vi "ScanMode_SLM.vi"() -> ()   [LabVIEW 2014]
uses:
  Controls/Scan_SLM.ctl
  Controls/MetricControl_SLM.ctl
  Controls/Scan Metric_SLM.ctl
  Controls/ScanEngineState_SLM.ctl
  <vilib>/Analysis/6fits.llb/Curve Fitting Criteria.ctl
  <vilib>/Utility/miscctls.llb/LVPointDoubleTypeDef.ctl
  <vilib>/Analysis/NI_AALPro.lvlib
  <vilib>/gmath/NI_Gmath.lvlib
panel:
  in  "Reset":bool
  out "Image":sgl[][](graph)
  in  "Apply":bool
  in  "Find peak":bool
  in  "Cancel":bool
  in  "Metric Control":T1
  in  "stop":bool
  out "Metric Display":cluster{"Amplititude":dbl[], "Metric":dbl[]}[](graph)
  in  "Scan Control":T3 {"Mode" items=["2", "3", "4", "5", "6", "7", "8", "9", "10", "11", "12", "13", "14", "15", "16", "17", "18", "19", "20", "21", "22", "23", "24", "25", "26", "27", "28", "29", "30", "31", "32", "33", "34", "35", "36", "37"]}
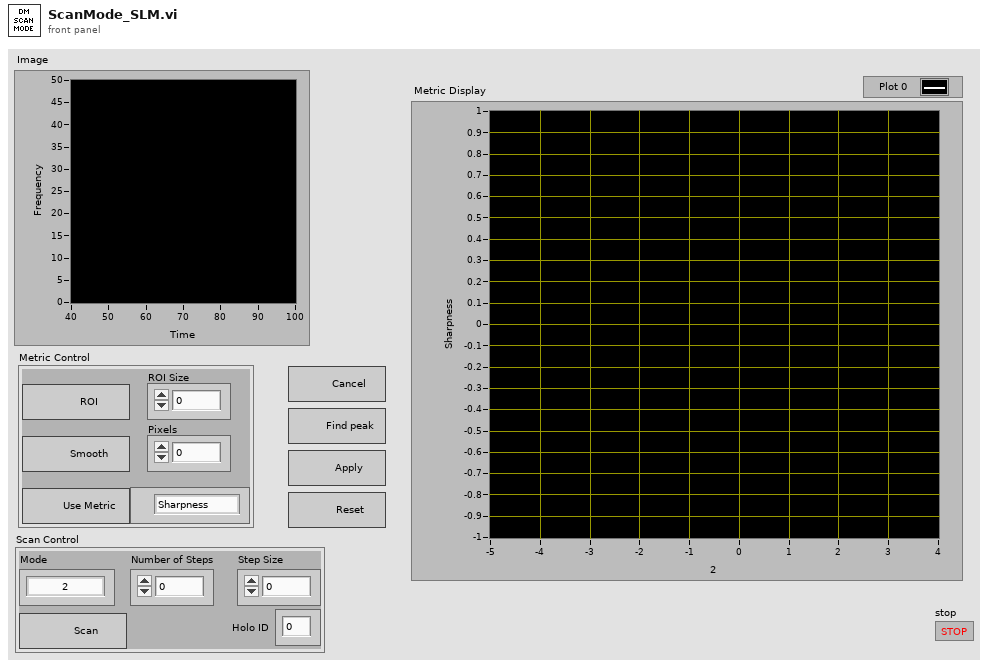
[diagram p1: front panel]
types:
  T1 = typedef "MetricControl_SLM.ctl" = cluster{"Use Metric":bool, "SLM Metric":T2, "Smooth":bool, "Pixels":dbl, "ROI":bool, "ROI Size":dbl}
  T2 = typedef "Scan Metric_SLM.ctl" = enum16{"Sharpness", "Brightness", "Combined"}
  T3 = typedef "Scan_SLM.ctl" = cluster{"Scan":bool, "Mode":u16, "Number of Steps":u8, "Step Size":dbl, "Holo ID":i32}
  T4 = typedef "ScanEngineState_SLM.ctl" = enum16{"SLM_WRITE", "IMAGE", ""}
  T5 = typedef "LVPointDoubleTypeDef.ctl" = cluster{"X":dbl, "Y":dbl}
  T6 = enum16{"Linear", "Polynomial", "Exponential", "Power"}
  T7 = typedef "Holo Settings.ctl" = cluster{"Top Hat":bool, "Modes":cluster{"Mode ID":string, "Amplititute":dbl}[], "Vortex":bool, "Clockwise":bool, "X":dbl, "Y":dbl, "Holo ON":bool, "Scan":bool}
  T8 = typedef "LVStringsAndValuesArrayTypeDef_U16.ctl" = cluster{"String":string, "Value":u16}[]
  T9 = typedef "NI_AALPro.lvlib/Curve Fitting Criteria.ctl" = u16
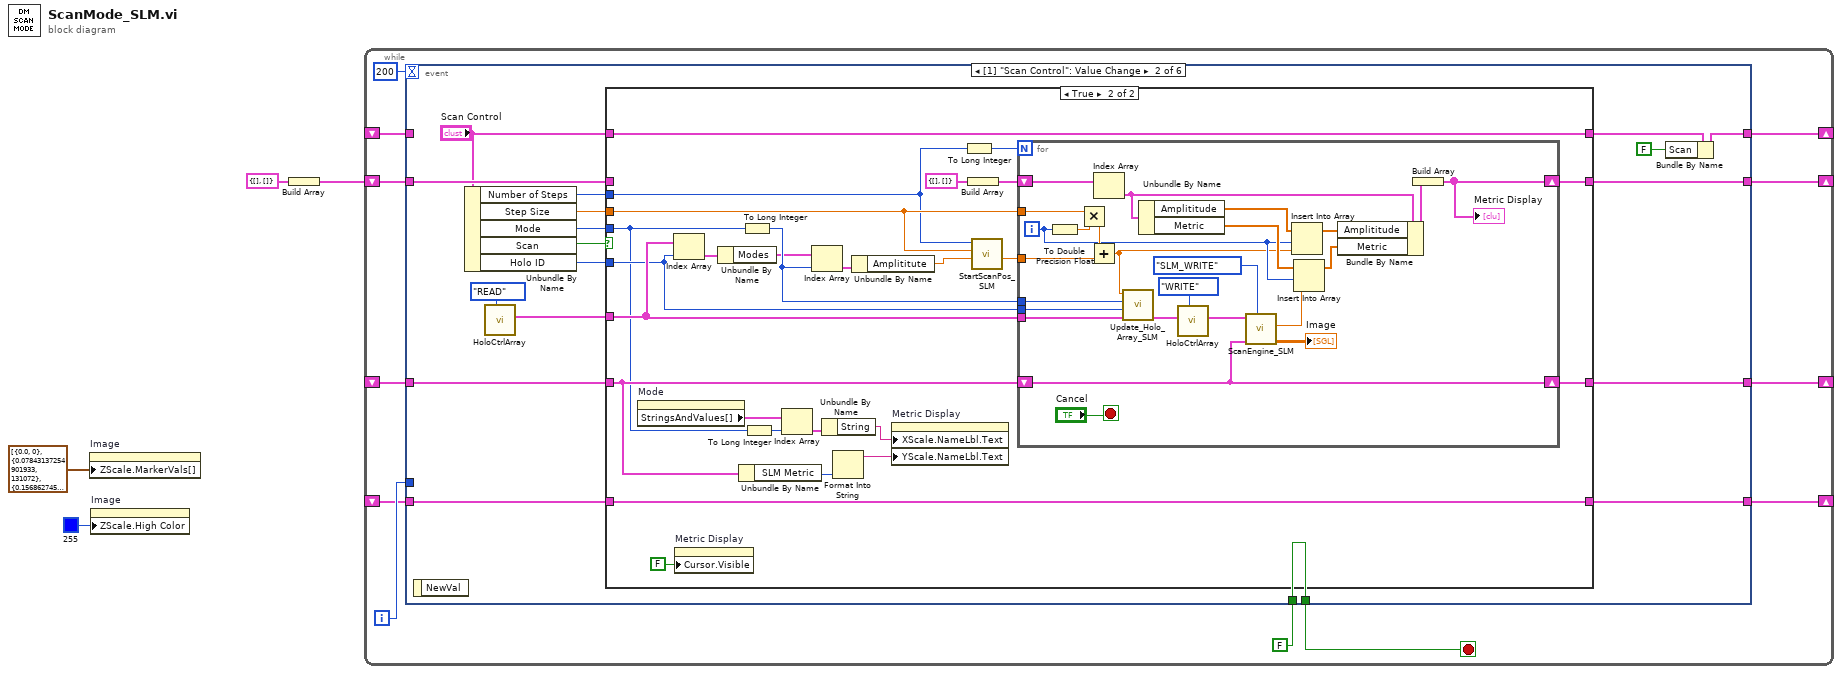
[diagram p0: block diagram]
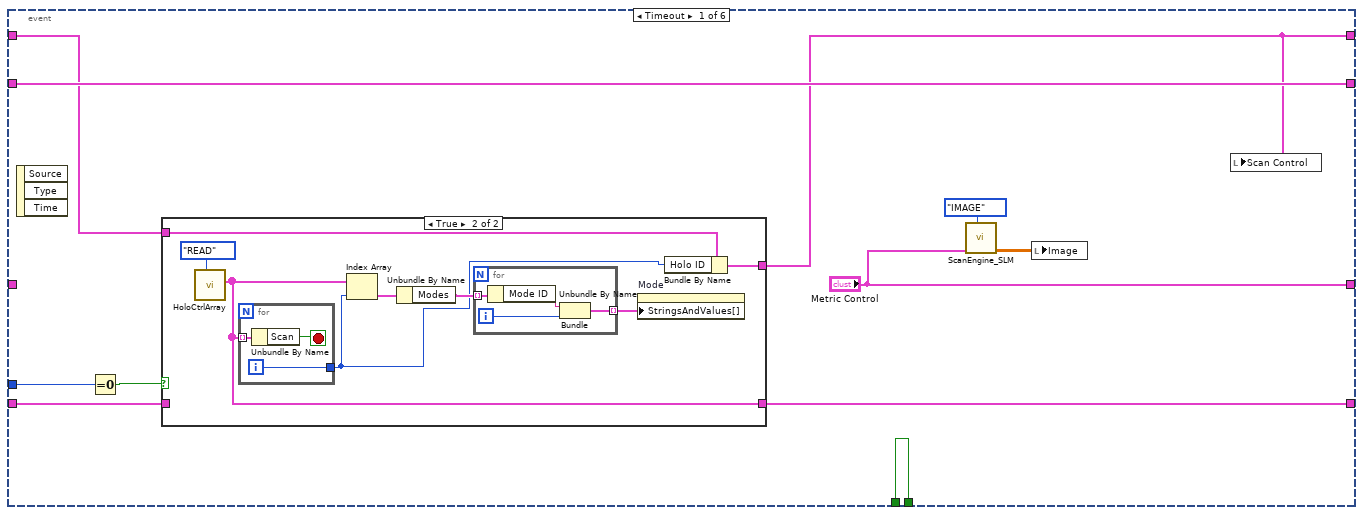
[diagram p2: hidden frame]
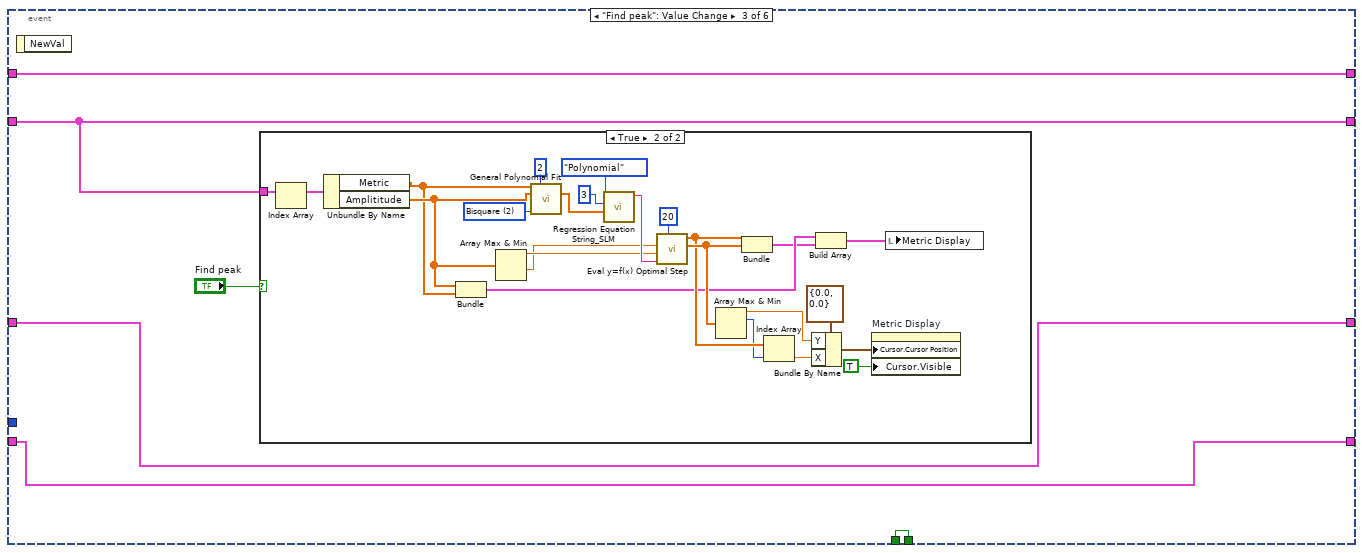
[diagram p5: hidden frame]
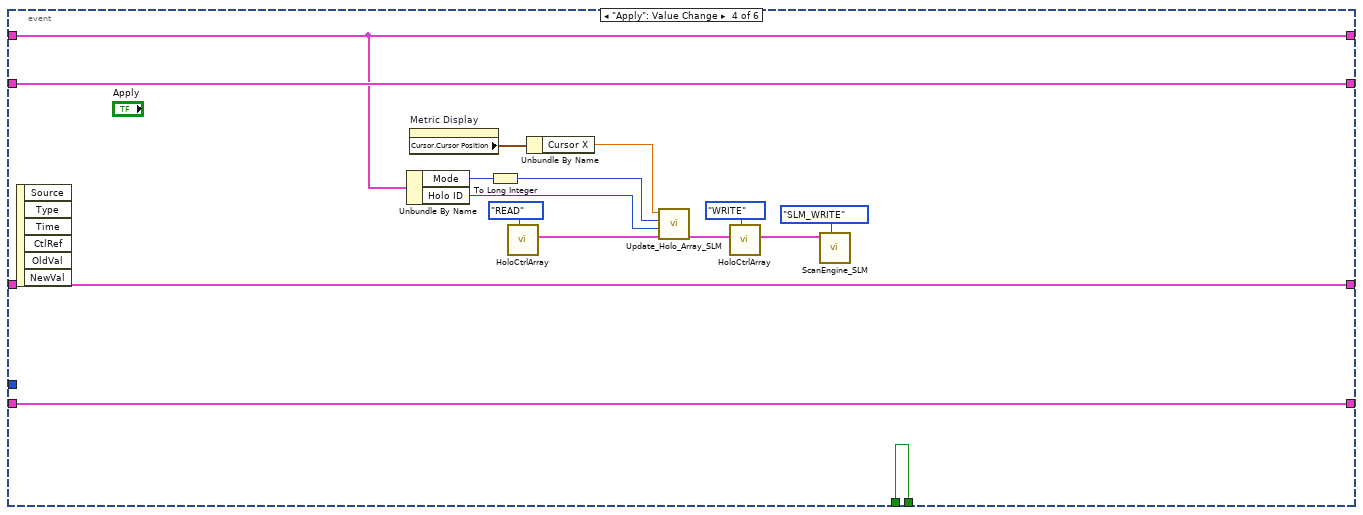
[diagram p7: hidden frame]
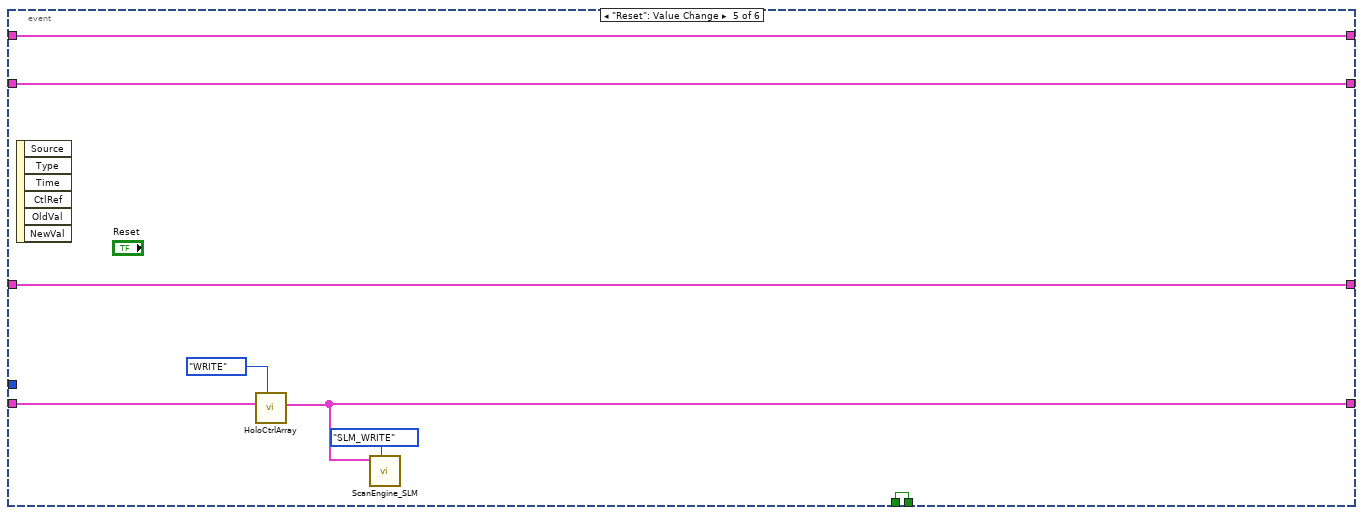
[diagram p8: hidden frame]
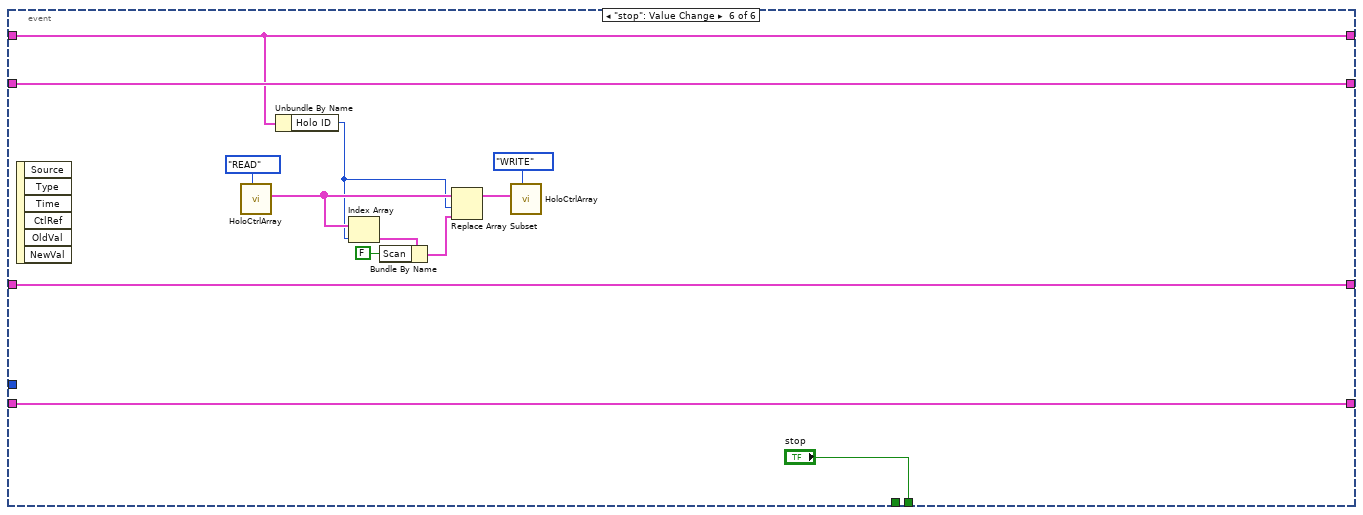
[diagram p9: hidden frame]
diagram:
  n1 = property on="Image" class="IntGraph (strict)"("ZScale.MarkerVals[]"=cluster{dbl, u32}[] [{0.0, 0}, {0.07843137254901933, 131072}, {0.15686274509805287, 196608}, {0.235294117647058, 327680}, {0.3137254901960773, 458752}, {0.39215686274509665, 589824}, {0.47058823529410176, 720896}, {0.5490196078431353, 851971}, {0.6274509803921546, 983043}, {0.705882352941174, 1114115}, {0.7843137254902075, 1245187}, {0.8627450980392268, 1376259}, {0.941176470588232, 1507331}, {1.0196078431372513, 1638403}, {1.0980392156862848, 1769475}, {1.1764705882353041, 1769479}, {1.2549019607843093, 2031623}, {1.3333333333333286, 2162695}, {1.4117647058823621, 2293767}, {1.4901960784313673, 2424839}, {1.5686274509803866, 2555911}, {1.647058823529406, 2686983}, {1.7254901960784395, 2818055}, {1.8039215686274588, 2949127}, {1.882352941176464, 3080203}, {1.9607843137254832, 3211275}, {2.0392156862745168, 3342347}, {2.117647058823522, 3473419}, {2.1960784313725554, 3604491}, {2.2745098039215605, 3735563}, {2.352941176470594, 3866635}, {2.431372549019599, 3867403}, {2.5098039215686327, 4129547}, {2.588235294117638, 4260619}, {2.6666666666666714, 4391691}, {2.7450980392156907, 4522763}, {2.823529411764696, 4653839}, {2.901960784313715, 4784911}, {2.9803921568627487, 4915983}, {3.058823529411768, 5178127}, {3.1372549019607874, 5309199}, {3.2156862745097925, 5440271}, {3.294117647058826, 5571343}, {3.3725490196078454, 5702415}, {3.4509803921568647, 5703439}, {3.52941176470587, 5965583}, {3.6078431372549034, 6096655}, {3.6862745098039227, 6227727}, {3.764705882352942, 6358799}, {3.8431372549019756, 6489871}, {3.9215686274509807, 6620943}, {4.0, 6752015}, {4.078431372549019, 6883087}, {4.1568627450980244, 7015183}, {4.235294117647058, 7146255}, {4.313725490196077, 7277327}, {4.392156862745097, 7408399}, {4.470588235294102, 7539471}, {4.549019607843135, 7670543}, {4.627450980392155, 7801615}, {4.705882352941174, 8063759}, {4.784313725490179, 8194831}, {4.862745098039213, 8326927}, {4.941176470588232, 8457999}, {5.019607843137251, 8589075}, {5.098039215686285, 8720147}, {5.17647058823529, 8851219}, {5.254901960784309, 8982291}, {5.333333333333329, 9113363}, {5.411764705882362, 9114387}, {5.490196078431367, 9376531}, {5.568627450980401, 9507603}, {5.647058823529406, 9638675}, {5.7254901960784395, 9769747}, {5.803921568627445, 9901843}, {5.882352941176478, 10032915}, {5.960784313725483, 10163987}, {6.039215686274517, 10229523}, {6.117647058823522, 10295059}, {6.196078431372555, 10427155}, {6.2745098039215605, 10558227}, {6.352941176470594, 10689299}, {6.431372549019599, 10820371}, {6.509803921568633, 10886931}, {6.588235294117638, 10952467}, {6.666666666666671, 11083539}, {6.745098039215691, 11214611}, {6.82352941176471, 11215635}, {6.901960784313715, 11477779}, {6.980392156862749, 11543315}, {7.058823529411768, 11608851}, {7.137254901960787, 11740947}, {7.215686274509821, 11806483}, {7.294117647058826, 11872019}, {7.372549019607845, 12004115}, {7.450980392156865, 12135187}, {7.529411764705898, 12266259}, {7.607843137254903, 12267283}, {7.686274509803923, 12398355}, {7.764705882352942, 12529427}, {7.843137254901947, 12530451}, {7.921568627450981, 12595987}, {8.0, 12530451}, {8.07843137254902, 12793619}, {8.156862745098024, 12794131}, {8.235294117647058, 12794643}, {8.313725490196077, 13056787}, {8.392156862745097, 13057299}, {8.47058823529413, 13057811}, {8.549019607843135, 13188883}, {8.627450980392155, 13320979}, {8.705882352941174, 13386515}, {8.784313725490179, 13452563}, {8.862745098039213, 13584147}, {8.941176470588232, 13584659}, {9.019607843137251, 13585171}, {9.098039215686256, 13585683}, {9.17647058823529, 13717267}, {9.254901960784323, 13848339}, {9.333333333333329, 13849363}, {9.411764705882362, 13849875}, {9.490196078431367, 13850387}, {9.5686274509804, 13981459}, {9.647058823529406, 14113555}, {9.72549019607844, 14114067}, {9.803921568627445, 14114579}, {9.882352941176478, 14115091}, {9.960784313725483, 14246675}, {10.039215686274517, 14377747}, {10.117647058823522, 14378771}, {10.196078431372555, 14379283}, {10.27450980392156, 14379539}, {10.352941176470594, 14379795}, {10.4313725490196, 14380819}, {10.509803921568633, 14511891}, {10.588235294117638, 14643987}, {10.666666666666671, 14644503}, {10.745098039215677, 14645015}, {10.82352941176471, 14645527}, {10.901960784313744, 14646039}, {10.980392156862749, 14646551}, {11.058823529411768, 14778135}, {11.137254901960787, 14909207}, {11.215686274509821, 14910231}, {11.294117647058826, 14910747}, {11.372549019607845, 14911259}, {11.450980392156865, 14911771}, {11.52941176470587, 14912283}, {11.607843137254903, 14912797}, {11.686274509803923, 15044383}, {11.764705882352942, 15175455}, {11.843137254901947, 15175967}, {11.92156862745098, 15176479}, {12.0, 15176991}, {12.07843137254902, 15177507}, {12.156862745098053, 15178019}, {12.235294117647058, 15178531}, {12.313725490196092, 15310115}, {12.392156862745097, 15441701}, {12.47058823529413, 15441959}, {12.549019607843135, 15442215}, {12.627450980392155, 15442727}, {12.705882352941174, 15443243}, {12.784313725490179, 15443755}, {12.862745098039213, 15444269}, {12.941176470588246, 15444783}, {13.019607843137251, 15444783}, {13.098039215686285, 15576367}, {13.17647058823529, 15707953}, {13.25490196078431, 15708467}, {13.333333333333329, 15708979}, {13.411764705882362, 15708981}, {13.490196078431367, 15708983}, {13.568627450980387, 15710011}, {13.647058823529406, 15710523}, {13.725490196078411, 15711037}, {13.803921568627459, 15711039}, {13.882352941176464, 15711553}, {13.960784313725512, 15843139}, {14.039215686274517, 15974213}, {14.117647058823522, 15974215}, {14.196078431372541, 15974217}, {14.27450980392156, 15974219}, {14.352941176470594, 15975755}, {14.431372549019613, 15976271}, {14.509803921568633, 15976785}, {14.588235294117666, 15977299}, {14.666666666666671, 15977301}, {14.745098039215677, 15977815}, {14.82352941176471, 15978327}, {14.901960784313744, 15978331}, {14.980392156862749, 16109917}, {15.058823529411768, 16241503}, {15.137254901960787, 16241505}, {15.215686274509792, 16242019}, {15.294117647058826, 16242535}, {15.372549019607845, 16242537}, {15.450980392156865, 16242539}, {15.529411764705898, 16243563}, {15.607843137254903, 16243567}, {15.686274509803908, 16244081}, {15.764705882352942, 16244595}, {15.843137254901947, 16244599}, {15.92156862745098, 16244601}, {16.0, 16244603}, {16.07843137254902, 16245627}, {16.156862745098024, 16245631}, {16.235294117647058, 16245633}, {16.313725490196077, 16246147}, {16.392156862745097, 16246663}, {16.47058823529413, 16377735}, {16.549019607843135, 16508811}, {16.62745098039217, 16508815}, {16.705882352941174, 16509839}, {16.78431372549018, 16509843}, {16.862745098039213, 16509845}, {16.941176470588232, 16509847}, {17.01960784313725, 16510361}, {17.098039215686256, 16510875}, {17.17647058823529, 16510879}, {17.25490196078431, 16510881}, {17.33333333333333, 16510883}, {17.411764705882362, 16511399}, {17.49019607843138, 16511911}, {17.568627450980387, 16511915}, {17.647058823529406, 16511917}, {17.72549019607844, 16511919}, {17.80392156862746, 16511923}, {17.882352941176464, 16512437}, {17.960784313725483, 16512951}, {18.03921568627449, 16512955}, {18.117647058823522, 16512957}, {18.19607843137254, 16512959}, {18.27450980392156, 16512961}, {18.352941176470594, 16512963}, {18.431372549019613, 16512967}, {18.509803921568633, 16513481}, {18.588235294117638, 16513995}, {18.66666666666667, 16513999}, {18.74509803921569, 16514001}, {18.82352941176471, 16514003}, {18.901960784313744, 16514005}, {18.98039215686275, 16514007}, {19.058823529411754, 16514011}, {19.137254901960787, 16514013}, {19.215686274509792, 16514015}, {19.294117647058826, 16514019}, {19.372549019607845, 16514021}, {19.450980392156865, 16514023}, {19.52941176470587, 16514027}, {19.607843137254918, 16514029}, {19.686274509803923, 16514031}, {19.764705882352942, 16514035}, {19.843137254901947, 16514037}, {19.921568627450995, 16514039}, {20.0, 16514043}] ("Z Scale.Marker Values[]")) -> ()  [unwired: 2 in, 2 out]
  n2 = property on="Image" class="IntGraph (strict)"("ZScale.High Color"=u32 255) -> ()  [unwired: 2 in, 2 out]
  n3 = Build Array(cluster{"Amplititude":dbl[], "Metric":dbl[]} {"Amplititude"=[], "Metric"=[]} ("output cluster")) -> (w3:cluster{"Amplititude":dbl[], "Metric":dbl[]}[])
  n4 = while {
    shift-right: [w12] -> _
    shift-left: _ -> [w11]
    shift-right: [w10] -> _
    shift-left: w3 -> [w9]
    shift-right: [w7] -> _
    shift-left: _ -> [w8]
    shift-right: [w6] -> _
    shift-left: _ -> [w5]
    i -> [w13]
    stop <- w16 stop-if-true
    n5 = event shown="[1] \"Scan Control\": Value Change" {
      selector: _ -> [_ _ _ _ _ _]
      dyn-events: _ -> [_ _ _ _ _ _]
      timeout: 200 -> [_ _ _ _ _ _]
      tunnel: [w27 w60 w120 w159 w171 "stop"] -> w16
      tunnel: FALSE -> [w27 w60 w120 w159 w171 _]
      tunnel: w13 -> [w25 _ _ _ _ _]
      tunnel: [w19 w52 w123 w161 w170 w178] -> w12
      tunnel: w11 -> [w20 _ w123 w161 w170 w178]
      tunnel: [w24 w58 w122 w163 w169 w183] -> w10
      tunnel: w9 -> [w24 w56 w122 w163 w169 w183]
      tunnel: w8 -> [_ w51 w119 w158 w168 w182]
      tunnel: ["Metric Control" w47 w119 w158 w168 w182] -> w7
      tunnel: [w22 w46 w118 w148 w164 w181] -> w6
      tunnel: w5 -> [w21 w45 w118 w148 w166 w181]
      event Timeout {
        n6 = event-data() -> ()  [unwired: 1 in, 3 out]
        n7 = Equal To 0?(x=w25) -> (x = 0?=w26:bool)
        n8 = case shown="True" w26 {
          tunnel: [w29 w34] -> w22
          tunnel: w21 -> [w29 _]
          tunnel: w20 -> [w28 w33]
          tunnel: [w28 w31] -> w19
          frame False {
          }
          frame True {
            n9 = call "HoloCtrlArray.vi"("Action"=enum16{"READ", "WRITE"}."READ") -> ("Holo Array Out"=w34:T7[])  [unwired: 10 in]
            n10 = for {
              tunnel: w34 -> [w40] mode=indexing
              tunnel: [w39] -> w32
              i -> [w39]
              stop <- w38 stop-if-true
              n11 = Unbundle By Name(w40) -> ("Scan"=w38:bool)
            }
            n12 = Index Array(array=w34, index=w32) -> (element=w36:T7)
            n13 = Unbundle By Name(w36) -> ("Modes"=w35:cluster{"Mode ID":string, "Amplititute":dbl}[])
            n14 = for {
              tunnel: w35 -> [w44] mode=indexing
              tunnel: [w41] -> w30 mode=indexing
              i -> [w42]
              n15 = Unbundle By Name(w44) -> ("Mode ID"=w43:string)
              n16 = Bundle("Mode ID"=w43, w42) -> (w41:cluster{"Mode ID":string, i32})  [unwired: 1 in]
            }
            n17 = property on="Mode" class="Ring (strict)"("StringsAndValues[]"=w30) -> ()  [unwired: 2 in, 2 out]
            n18 = Bundle By Name(cluster=w33, "Holo ID"=w32) -> (w31:T3)
          }
        }
        n19 = call "ScanEngine_SLM.vi"("Action"=ScanEngineState_SLM."IMAGE", "Metric Control"="Metric Control") -> ("Metric Image"=w18:sgl[][])  [unwired: 8 in, 1 out]
        n20 = local write "Image"(w18) -> ()
        n21 = local write "Scan Control"(w19) -> ()
      }
      event Value Change {
        n22 = event-data() -> ()  [unwired: 1 in, 1 out]
        n23 = Unbundle By Name("Scan Control") -> ("Number of Steps"=w62:u8, "Step Size"=w61:dbl, "Mode"=w59:u16, "Scan"=w57:bool, "Holo ID"=w49:i32)
        n24 = call "HoloCtrlArray.vi"("Action"=enum16{"READ", "WRITE"}."READ") -> ("Holo Array Out"=w48:T7[])  [unwired: 10 in]
        n25 = case shown="True" w57 {
          tunnel: w62 -> [_ w73]
          tunnel: w61 -> [_ w92]
          tunnel: w59 -> [_ w69]
          tunnel: [w66 w81] -> w58
          tunnel: w56 -> [w66 _]
          tunnel: [w65 w85] -> w53
          tunnel: "Scan Control" -> [w65 w85]
          tunnel: w51 -> [w64 w80]
          tunnel: w49 -> [_ w76]
          tunnel: w48 -> [_ w77]
          tunnel: [w64 w75] -> w47
          tunnel: [w63 w72] -> w46
          tunnel: w45 -> [w63 w72]
          frame False {
          }
          frame True {
            n26 = property on="Mode" class="Ring (strict)"() -> ("StringsAndValues[]"=w71:T8)  [unwired: 2 in, 2 out]
            n27 = Index Array(array=w77, index=w76) -> (element=w78:T7)
            n28 = property on="Metric Display" class="XYGraph (strict)"("Cursor.Visible"=FALSE) -> ()  [unwired: 2 in, 2 out]
            n29 = Unbundle By Name(w78) -> ("Modes"=w79:cluster{"Mode ID":string, "Amplititute":dbl}[])
            n30 = Unbundle By Name(w80) -> ("SLM Metric"=w86:T2)
            n31 = To Long Integer(number=w69) -> (32bit integer=w89:i32)
            n32 = To Long Integer(number=w69) -> (32bit integer=w67:i32)
            n33 = Index Array(array=w71, index=w67) -> (element=w70:cluster{"String":string, "Value":u16})
            n34 = Index Array(array=w79, index=w89) -> (element=w90:cluster{"Mode ID":string, "Amplititute":dbl})
            n35 = Unbundle By Name(w70) -> ("String"=w68:string)
            n36 = Format Into String(w86) -> (resulting string=w87:string)  [unwired: 3 in, 1 out]
            n37 = Unbundle By Name(w90) -> ("Amplititute"=w91:dbl)
            n38 = property on="Metric Display" class="XYGraph (strict)"("XScale.NameLbl.Text"=w68, "YScale.NameLbl.Text"=w87) -> ()  [unwired: 2 in, 2 out]
            n39 = To Long Integer(number=w73) -> (32bit integer=w88:i32)
            n40 = Build Array(cluster{"Amplititude":dbl[], "Metric":dbl[]} {"Amplititude"=[], "Metric"=[]} ("output cluster")) -> (w82:cluster{"Amplititude":dbl[], "Metric":dbl[]}[])
            n41 = call "StartScanPos_SLM.vi"("Amplititute"=w91, "Step Size"=w92, "Number of Steps"=w73) -> ("Start Scan Position"=w74:dbl)  [unwired: 8 in]
            n42 = for {
              N: w88 -> [_]
              tunnel: w92 -> [w117]
              tunnel: w89 -> [w98]
              shift-right: [w104] -> w81
              shift-left: w82 -> [w113]
              tunnel: w77 -> [w96]
              tunnel: w76 -> [w97]
              shift-right: [w101] -> w75
              shift-left: w80 -> [w101]
              tunnel: w74 -> [w94]
              i -> [w110]
              stop <- "Cancel" stop-if-true
              n43 = To Double Precision Float(number=w110) -> (double precision float=w116:dbl)
              n44 = Multiply(x=w117, y=w116) -> (x*y=w115:dbl)
              n45 = Add(x=w115, y=w94) -> (x+y=w99:dbl)
              n46 = Index Array(array=w113) -> (element=w108:cluster{"Amplititude":dbl[], "Metric":dbl[]})  [unwired: 1 in]
              n47 = call "Update_Holo_Array_SLM.vi"("Holo Array In"=w96, "Holo ID"=w97, "Mode ID"=w98, "Amplititute"=w99) -> ("Update Holo Array"=w95:T7[])  [unwired: 7 in]
              n48 = Unbundle By Name(w108) -> ("Amplititude"=w112:dbl[], "Metric"=w111:dbl[])
              n49 = call "HoloCtrlArray.vi"("Action"=enum16{"READ", "WRITE"}."WRITE", "Holo Array In"=w95) -> ("Holo Array Out"=w100:T7[])  [unwired: 9 in]
              n50 = call "ScanEngine_SLM.vi"("Action"=ScanEngineState_SLM."SLM_WRITE", "Metric Control"=w101, "Holo Array In"=w100) -> ("Metric Image"=→"Image":sgl[][], "Metric Result"=w109:dbl)  [unwired: 7 in]
              n51 = Insert Into Array(array=w112, index=w110, new element=w99) -> (w107:dbl[])
              n52 = Insert Into Array(array=w111, index=w110, new element=w109) -> (w106:dbl[])
              n53 = Bundle By Name(cluster=w108, "Amplititude"=w107, "Metric"=w106) -> (w105:cluster{"Amplititude":dbl[], "Metric":dbl[]})
              n54 = Build Array(w105) -> (w104:cluster{"Amplititude":dbl[], "Metric":dbl[]}[])
              "Metric Display" <- w104
            }
          }
        }
        n55 = Bundle By Name(cluster=w53, "Scan"=FALSE) -> (w52:T3)
      }
      event "Find peak": Value Change {
        n56 = event-data() -> ()  [unwired: 1 in, 1 out]
        n57 = case shown="True" "Find peak" {
          tunnel: w122 -> [_ w128]
          frame False {
          }
          frame True {
            w147 = T9 2 items=["Least Square", "Least Absolute Residual", "Bisquare"] ("method")
            n58 = Index Array(array=w128) -> (element=w127:cluster{"Amplititude":dbl[], "Metric":dbl[]})  [unwired: 1 in]
            n59 = Unbundle By Name(w127) -> ("Metric"=w124:dbl[], "Amplititude"=w130:dbl[])
            n60 = Bundle("Amplititude"=w130, "Metric"=w124) -> (w126:cluster{"Amplititude":dbl[], "Metric":dbl[]})  [unwired: 1 in]
            n61 = Array Max & Min(array=w130) -> (max value=w140:dbl, min value=w139:dbl)  [unwired: 2 out]
            n62 = call <vilib>:"General Polynomial Fit.vi"("Y"=w124, "polynomial order"=2, "X"=w130, "method"=w147) -> ("Polynomial Coefficients"=w144:dbl[])  [unwired: 8 in, 3 out]
            n63 = call "Regression Equation String_SLM.vi"("coefficients"=w144, "precision"=3, "fit type"=T6."Polynomial") -> ("Formula"=w142:string)  [unwired: 8 in]
            n64 = call <vilib>:"Eval y=f(x) Optimal Step.vi"("number of points"=u32 20, "formula"=w142, "end"=w140, "start"=w139) -> ("Y Values"=w138:dbl[], "X Values"=w137:dbl[])  [unwired: 1 in, 2 out]
            n65 = Array Max & Min(array=w138) -> (max value=w134:dbl, max index (indices)=w136:i32)  [unwired: 2 out]
            n66 = Bundle("X Values"=w137, "Y Values"=w138) -> (w125:cluster{"X Values":dbl[], "Y Values":dbl[]})  [unwired: 1 in]
            n67 = Index Array(array=w137, index=w136) -> (element=w133:dbl)
            n68 = Bundle By Name(cluster=T5 {"X"=0.0, "Y"=0.0} ("Cursor.Cursor Position"), "Y"=w134, "X"=w133) -> (w132:T5)
            n69 = Build Array(w126, w125) -> (w129:cluster{"X Values":dbl[], "Y Values":dbl[]}[])
            n70 = property on="Metric Display" class="XYGraph (strict)"("Cursor.Cursor Position"=w132, "Cursor.Visible"=TRUE) -> ()  [unwired: 2 in, 2 out]
            n71 = local write "Metric Display"(w129) -> ()
          }
        }
      }
      event "Apply": Value Change {
        n72 = event-data() -> ()  [unwired: 1 in, 6 out]
        n73 = Unbundle By Name(w161) -> ("Mode"=w160:u16, "Holo ID"=w155:i32)
        n74 = property on="Metric Display" class="XYGraph (strict)"() -> ("Cursor.Cursor Position"=w162:T5)  [unwired: 2 in, 2 out]
        n75 = To Long Integer(number=w160) -> (32bit integer=w156:i32)
        n76 = call "HoloCtrlArray.vi"("Action"=enum16{"READ", "WRITE"}."READ") -> ("Holo Array Out"=w154:T7[])  [unwired: 10 in]
        n77 = Unbundle By Name(w162) -> ("Cursor X"=w157:dbl)
        n78 = call "Update_Holo_Array_SLM.vi"("Holo Array In"=w154, "Holo ID"=w155, "Mode ID"=w156, "Amplititute"=w157) -> ("Update Holo Array"=w151:T7[])  [unwired: 7 in]
        n79 = call "HoloCtrlArray.vi"("Action"=enum16{"READ", "WRITE"}."WRITE", "Holo Array In"=w151) -> ("Holo Array Out"=w150:T7[])  [unwired: 9 in]
        n80 = call "ScanEngine_SLM.vi"("Action"=ScanEngineState_SLM."SLM_WRITE", "Holo Array In"=w150) -> ()  [unwired: 8 in, 2 out]
      }
      event "Reset": Value Change {
        n81 = event-data() -> ()  [unwired: 1 in, 6 out]
        n82 = call "HoloCtrlArray.vi"("Action"=enum16{"READ", "WRITE"}."WRITE", "Holo Array In"=w166) -> ("Holo Array Out"=w164:T7[])  [unwired: 9 in]
        n83 = call "ScanEngine_SLM.vi"("Action"=ScanEngineState_SLM."SLM_WRITE", "Holo Array In"=w164) -> ()  [unwired: 8 in, 2 out]
      }
      event "stop": Value Change {
        n84 = event-data() -> ()  [unwired: 1 in, 6 out]
        n85 = call "HoloCtrlArray.vi"("Action"=enum16{"READ", "WRITE"}."READ") -> ("Holo Array Out"=w174:T7[])  [unwired: 10 in]
        n86 = Unbundle By Name(w178) -> ("Holo ID"=w173:i32)
        n87 = Index Array(array=w174, index=w173) -> (element=w177:T7)
        n88 = Bundle By Name(cluster=w177, "Scan"=FALSE) -> (w175:T7)
        n89 = Replace Array Subset(array=w174, new element=w175, index=w173) -> (w172:T7[])
        n90 = call "HoloCtrlArray.vi"("Action"=enum16{"READ", "WRITE"}."WRITE", "Holo Array In"=w172) -> ()  [unwired: 9 in, 1 out]
      }
    }
  }
